vi "setUp.vi"(8 "error in":errorcluster, 11 "reference in":refnum<class "AIM ARINC 664 Loopback-SingleDevice.lvclass">=refnum) -> (0 "error out":errorcluster, 3 "reference out":refnum<class "AIM ARINC 664 Loopback-SingleDevice.lvclass">)   [LabVIEW 2020, in "AIM ARINC 664 Loopback-SingleDevice.lvclass"]
doc: "setUp runs prior to the test method during test execution. Use this method to initialize any object data required by your tests."
uses:
  AIM ARINC 664 Loopback-SingleDevice.lvclass
  C:/Program Files/National Instruments/LabVIEW 2024/vi.lib/addons/_JKI Toolkits/VI Tester/TestCase.llb/TestCase.lvclass
  AIM ARINC 664 Loopback-SingleDevice.lvclass/AIM ARINC 664 Loopback-SingleDevice.ctl
  <vilib>/addons/_JKI Toolkits/VI Tester/TestCase.llb/TestCase.lvclass
panel:
  in  "iterations":i32=2
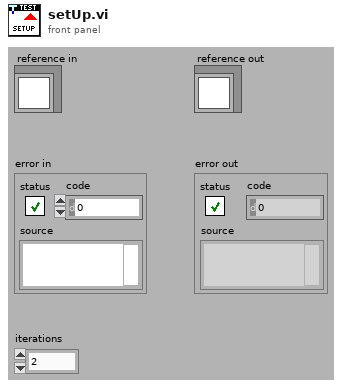
[diagram p1: front panel]
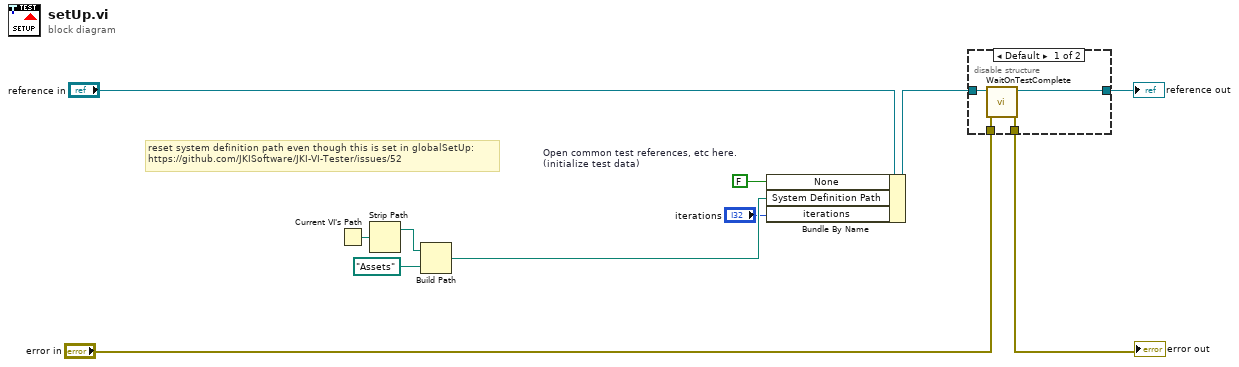
[diagram p0: block diagram]
diagram:
  w6 = FALSE  # Open common test references, etc here. (initialize test data)
  # "reset system definition path even though this is set in globalSetUp:\nhttps://github.com/JKISoftware/JKI-VI-Tester/issues/52"
  n1 = Current VI's Path() -> (path=w3:path)
  n2 = Strip Path(path=w3) -> (stripped path=w4:path)  [unwired: 1 out]
  n3 = Build Path(base path=w4, name or relative path=path "Assets" ("System Definition Name")) -> (appended path=w2:path)
  n4 = Bundle By Name(cluster="reference in", "None"=w6, "System Definition Path"=w2, "iterations"="iterations") -> (w7:refnum<class "AIM ARINC 664 Loopback-SingleDevice.lvclass">)
  n5 = disable-structure shown="Default" {
    disable-tunnel: "error in" -> [w15 w16]
    disable-tunnel: [w14 w16] -> w10
    disable-tunnel: [w13 w17] -> w8
    disable-tunnel: w7 -> [w12 w17]
    frame condition #0 (active) {
      n6 = call <vilib>:"WaitOnTestComplete.vi"("error in (no error)"=w15, "TestCase in"=w12) -> ("error out"=w14:errorcluster, "TestCase out"=w13:refnum<class "AIM ARINC 664 Loopback-SingleDevice.lvclass">)  [unwired: 8 in]
    }
    frame condition #1 {
    }
  }
  "error out" <- w10
  "reference out" <- w8
